vi "Messenger hub.vi"() -> ()   [LabVIEW 2021, in "Queued messenger.lvlib"]
doc: "Example of messenger that receives messages from other modules and distributes them to recipients."
uses:
  <userlib>/MatS libs/MatS Messenger/Queued messenger.lvlib
  <userlib>/MatS libs/MatS Messenger/TypeDefs/General message.ctl
  <userlib>/MatS libs/MatS Messenger/TypeDefs/Mailbox ref.ctl
  <userlib>/MatS libs/MatS Messenger/TypeDefs/Mailboxes.ctl
panel:
  in  "Master module":string
  in  "Supervisor":T1
  out "pending messages":i32
  in  "Mailboxes":T2
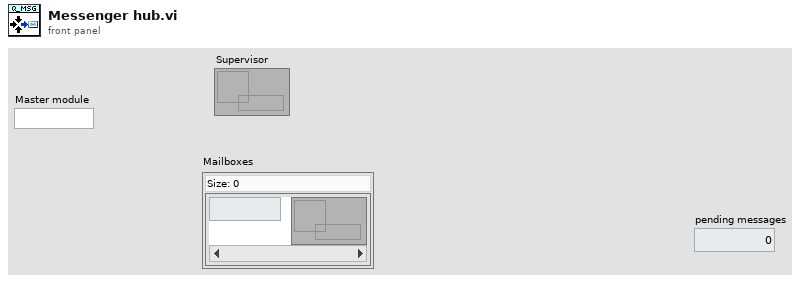
[diagram p1: front panel]
types:
  T1 = typedef "Queued messenger.lvlib/Mailbox ref.ctl" = refnum<queue>
  T2 = typedef "Queued messenger.lvlib/Mailboxes.ctl" = map{string, T1}
  T3 = typedef "Queued messenger.lvlib/General message.ctl" = cluster{"Sender":string, "Recipient":string, "Topic":string, "Content":variant, "Time Stamp":timestamp}
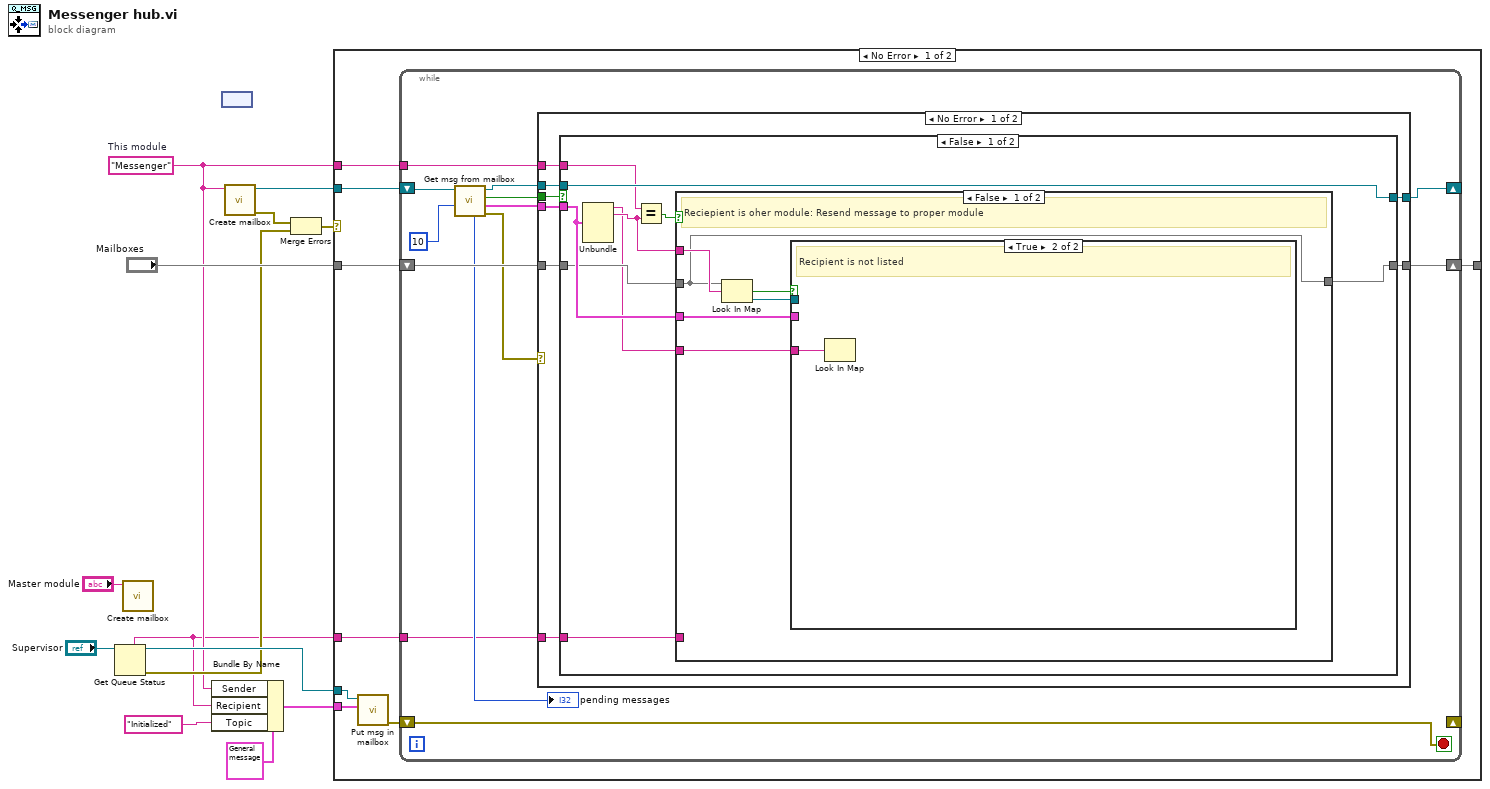
[diagram p0: block diagram]
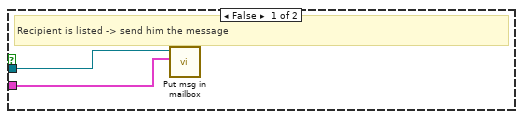
[diagram p2: hidden frame]
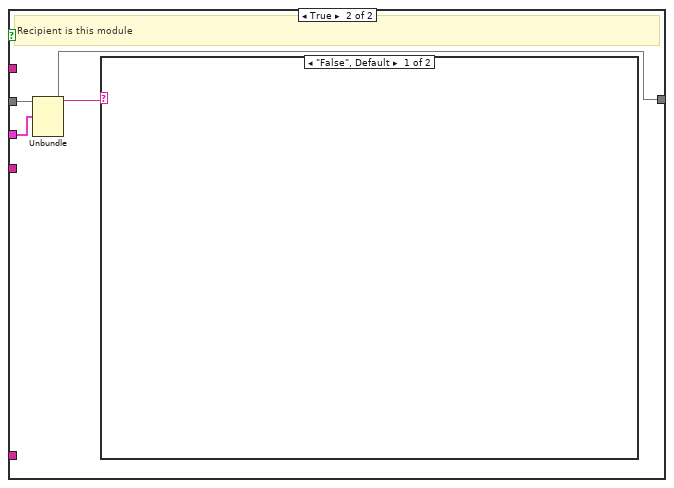
[diagram p3: hidden frame]
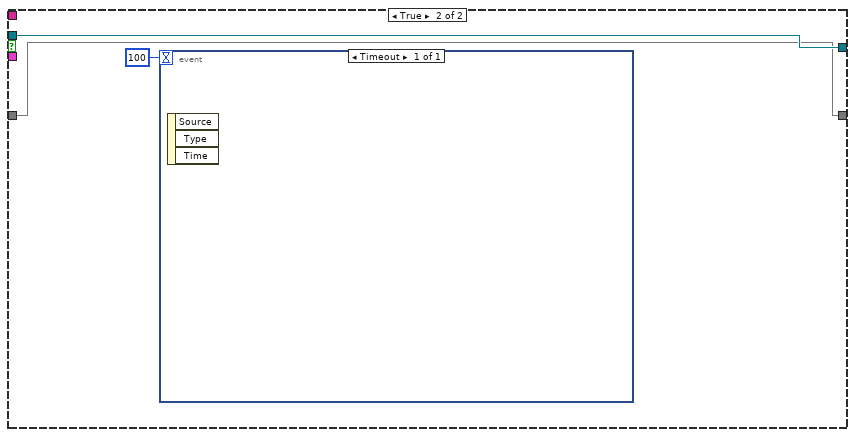
[diagram p5: hidden frame]
diagram:
  w3 = "Messenger"  # This module
  n1 = Get Queue Status(queue="Supervisor") -> (queue out=w6:T1, queue name=w2:string, error out=w4:errorcluster)  [unwired: 2 in, 5 out]
  n2 = call <userlib>:"Create mailbox.vi"("name (unnamed)"="Master module") -> ()  [unwired: 4 in, 3 out]
  n3 = Bundle By Name(cluster=T3 {"Sender"="Messenger", "Recipient"="Supervisor", "Topic"="", "Content"=variant, "Time Stamp"=timestamp(0 s since 1904-01-01)} ("Message"), "Sender"=w3, "Recipient"=w2, "Topic"="Initialized") -> (w7:T3)
  n4 = node() -> ()  [unwired: 2 in, 1 out]
  n5 = call <userlib>:"Create mailbox.vi"("name (unnamed)"=w3) -> ("error out"=w12:errorcluster, "Mailbox ref"=w13:T1)  [unwired: 4 in, 1 out]
  n6 = Merge Errors(w12, w4) -> (w5:errorcluster)
  n7 = case shown="No Error" w5 {
    tunnel: w13 -> [w21 _]
    tunnel: "Mailboxes" -> [w20 _]
    tunnel: [w19 _] -> _
    tunnel: w7 -> [w18 _]
    tunnel: w6 -> [w17 _]
    tunnel: w3 -> [w15 _]
    tunnel: w2 -> [w14 _]
    frame No Error {
      n8 = call <userlib>:"Put msg in mailbox.vi"("Message"=w18, "Mailbox ref in"=w17) -> ("error out"=w16:errorcluster)  [unwired: 7 in, 2 out]
      n9 = while {
        shift-right: [w25] -> _
        shift-left: w21 -> [w34]
        shift-right: _ -> [_]
        shift-left: w16 -> [w24]
        tunnel: w15 -> [w23]
        tunnel: w14 -> [w22]
        shift-right: [w31] -> w19
        shift-left: w20 -> [w32]
        stop <- w24 stop-if-true
        n10 = call <userlib>:"Get msg from mailbox.vi"("timeout ms (1000)"=10, "Mailbox ref in"=w34) -> ("error out"=w30:errorcluster, "Message"=w27:T3, "timed out?"=w29:bool, "mailbox ref out"=w26:T1, "pending messages"=→"pending messages":i32)  [unwired: 4 in, 1 out]
        n11 = case shown="No Error" w30 {
          tunnel: w32 -> [w42 w67]
          tunnel: [w41 w67] -> w31
          tunnel: w29 -> [w40 _]
          tunnel: w27 -> [w39 _]
          tunnel: w26 -> [w38 w68]
          tunnel: [w37 w68] -> w25
          tunnel: w23 -> [w36 _]
          tunnel: w22 -> [w35 _]
          frame No Error {
            n12 = case shown="False" w40 {
              tunnel: w42 -> [w49 w64]
              tunnel: [w48 w64] -> w41
              tunnel: w39 -> [w50 _]
              tunnel: [w51 w65] -> w37
              tunnel: w38 -> [w51 w65]
              tunnel: w36 -> [w46 _]
              tunnel: w35 -> [w44 _]
              frame False {
                n13 = Unbundle(w50) -> ("Sender"=w43:string, "Recipient"=w45:string)  [unwired: 3 out]
                n14 = Equal?(x=w46, y=w45) -> (x = y?=w47:bool)
                n15 = case shown="False" w47 {
                  tunnel: w50 -> [w55 w63]
                  tunnel: w49 -> [w53 w61]
                  tunnel: [w53 w61] -> w48
                  tunnel: w45 -> [w54 _]
                  tunnel: w44 -> [_ _]
                  tunnel: w43 -> [w52 _]
                  frame False {
                    # "Reciepient is oher module: Resend message to proper module"
                    n16 = Look In Map(map=w53, key=w54) -> (key not found?=w57:bool, value=w56:T1)  [unwired: 1 in]
                    n17 = case shown="True" w57 {
                      tunnel: w56 -> [w59 _]
                      tunnel: w55 -> [w58 _]
                      tunnel: w52 -> [_ w60]
                      frame False {
                        # "Recipient is listed -> send him the message"
                        n18 = call <userlib>:"Put msg in mailbox.vi"("Message"=w58, "Mailbox ref in"=w59) -> ()  [unwired: 7 in, 3 out]
                      }
                      frame True {
                        # "Recipient is not listed"
                        n19 = Look In Map(key=w60) -> ()  [unwired: 2 in, 2 out]
                      }
                    }
                  }
                  frame True {
                    # "Recipient is this module"
                    n20 = Unbundle(w63) -> ("Sender"=w62:string)  [unwired: 4 out]
                    n21 = case shown="\"False\", Default" w62 {
                      frame "False", Default {
                      }
                      frame "True" {
                      }
                    }
                  }
                }
              }
              frame True {
                n22 = event shown="[0] Timeout" {
                  selector: _ -> [_]
                  dyn-events: _ -> [_]
                  timeout: 100 -> [_]
                  event Timeout {
                    n23 = event-data() -> ()  [unwired: 1 in, 3 out]
                  }
                }
              }
            }
          }
          frame Error {
          }
        }
      }
    }
    frame Error {
    }
  }
